vi "channelcontrolsub.vi"(0 "TorqueSample":dbl, 1 "dt":dbl, 3 "Limit Number":dbl, 4 "Torque":bool, 5 "ControlPara":dbl[](array[numeric]), 7 "AngleSample":dbl, 8 "Angel":bool, 9 "syn-Error":dbl, 12 "Command":dbl, 15 "TempAngle":dbl, 16 "output range":cluster{"output high":dbl, "output low":dbl}, 17 "ChannelStatus":T1 items=["通道关", "位置通道", "加载通道"]) -> (19 "syn out":dbl, 20 "output":dbl, 22 "forward":dbl, 23 "TempAngleOut":dbl, 24 "diff syn out 2":dbl, 25 "control out":dbl, 27 "Commandout":dbl)   [LabVIEW 2014]
uses:
  Control 1.ctl
  <vilib>/Analysis/3filter.llb/Filter Passband Type.ctl
  <vilib>/addons/control/pid/pid.llb/PID (DBL).vi
  <vilib>/addons/control/pid/NI_PID_pid.lvlib
  <vilib>/ptbypt/NI_PtbyPt.lvlib
  <vilib>/Analysis/NI_AALBase.lvlib
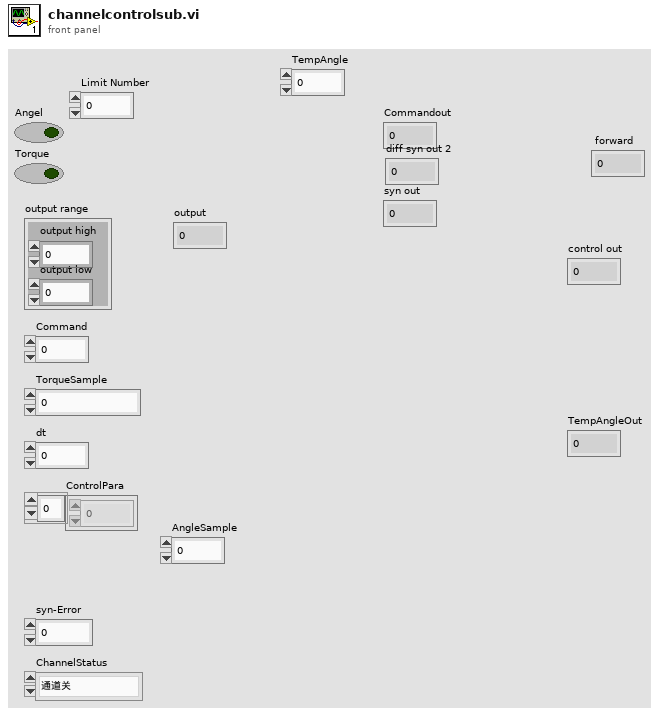
[diagram p1: front panel]
types:
  T1 = typedef "Control 1.ctl" = i32
  T2 = typedef "NI_AALBase.lvlib/Filter Passband Type.ctl" = enum32{"Lowpass", "Highpass", "Bandpass", "Bandstop"}
  T3 = cluster{"Numeric":dbl, "Numeric":dbl, "Numeric":dbl}
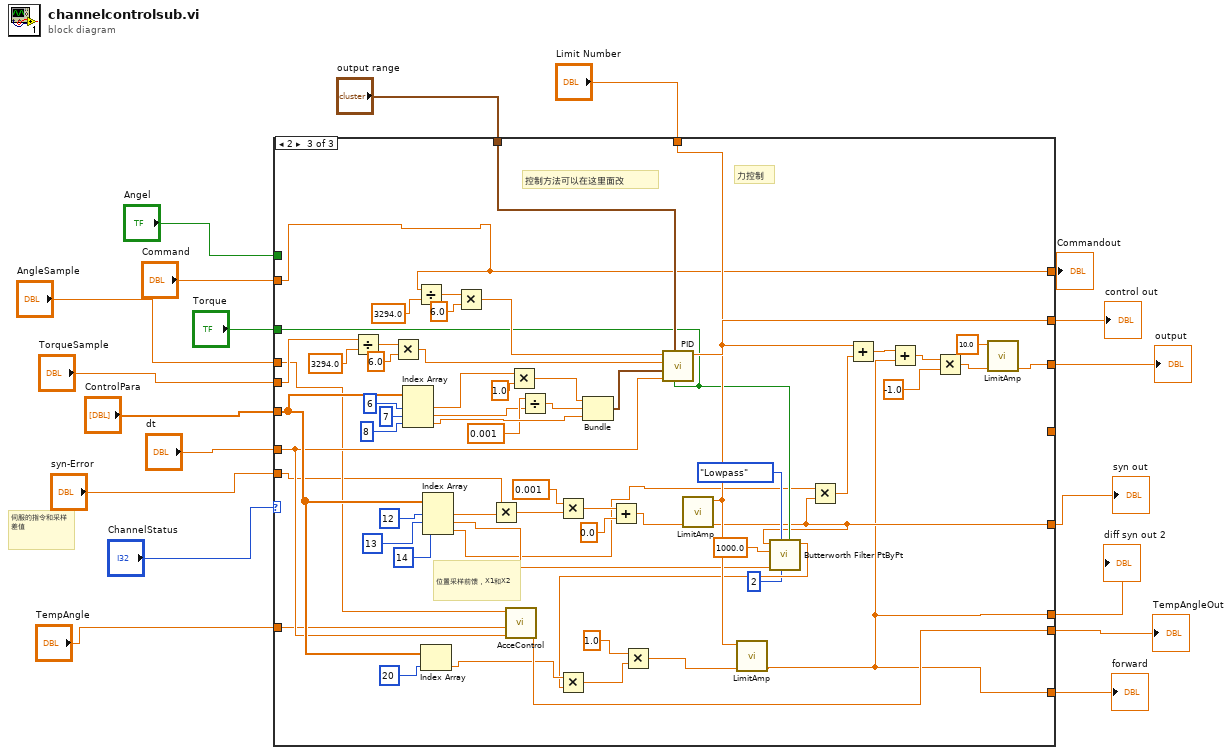
[diagram p0: block diagram]
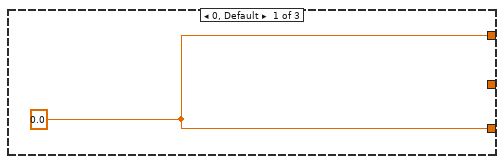
[diagram p2: hidden frame]
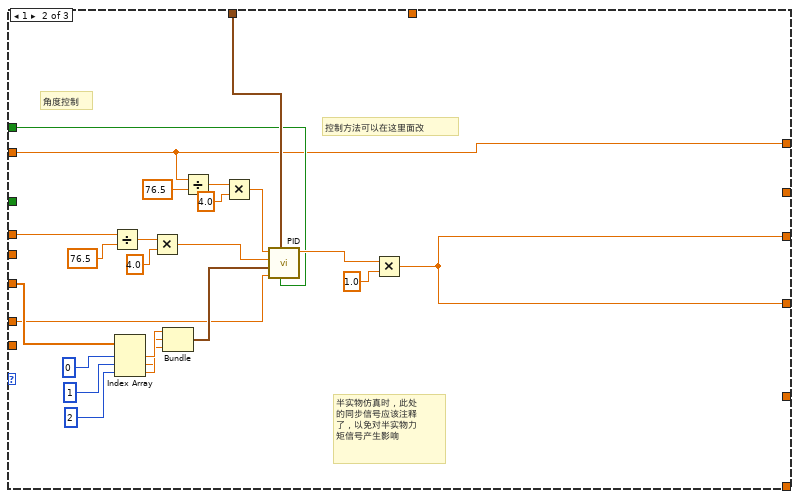
[diagram p3: hidden frame]
diagram:
  # "伺服的指令和采样差值"
  n1 = case shown="2" "ChannelStatus" {
    tunnel: "dt" -> [_ w29 w71]
    tunnel: "output range" -> [_ w26 w104]
    tunnel: "Command" -> [_ w21 w68]
    tunnel: "ControlPara" -> [_ w41 w80]
    tunnel: [w20 w24 w48] -> w18
    tunnel: "TorqueSample" -> [_ _ w89]
    tunnel: "syn-Error" -> [_ _ w67]
    tunnel: [_ w24 _] -> _
    tunnel: "AngleSample" -> [_ w23 w70]
    tunnel: "Angel" -> [_ w22 _]
    tunnel: "Torque" -> [_ _ w60]
    tunnel: [w20 w21 w68] -> w9
    tunnel: "TempAngle" -> [_ _ w69]
    tunnel: [_ _ w85] -> w8
    tunnel: [_ _ w82] -> w7
    tunnel: "Limit Number" -> [_ _ w78]
    tunnel: [_ _ w52] -> w2
    tunnel: [_ _ w46] -> w1
    tunnel: [_ _ w46] -> w5
    frame 0, Default {
      w20 = 0.0 ("output")
    }
    frame 1 {
      # "半实物仿真时，此处\n的同步信号应该注释\n了，以免对半实物力\n矩信号产生影响"
      # "控制方法可以在这里面改"
      # "角度控制"
      n2 = Divide(x=w23, y=76.5) -> (x/y=w35:dbl)
      n3 = Index Array(array=w41, index #1=0 ("index"), index #2=1 ("index"), index #3=2 ("index")) -> (element #1=w33:dbl, element #2=w25:dbl, element #3=w32:dbl)
      n4 = Multiply(x=w35, y=4.0) -> (x*y=w28:dbl)
      n5 = Bundle("Numeric"=w33, "Numeric"=w25, "Numeric"=w32) -> (w30:T3)  [unwired: 1 in]
      n6 = Divide(x=w21, y=76.5) -> (x/y=w38:dbl)
      n7 = Multiply(x=w38, y=4.0) -> (x*y=w27:dbl)
      n8 = call-poly <vilib>:"PID.vi"("reinitialize? (F)"=w22, "output range"=w26, "dt (s)"=w29, "PID gains"=w30, "process variable"=w28, "setpoint"=w27) -> ("output"=w31:dbl)  [unwired: 4 in, 1 out]
      n9 = Multiply(x=w31, y=1.0) -> (x*y=w24:dbl)
    }
    frame 2 {
      # "位置采样前馈，X1和X2"
      # "力控制"
      # "控制方法可以在这里面改"
      n10 = Divide(x=w89, y=3294.0) -> (x/y=w93:dbl)
      n11 = Multiply(x=w93, y=6.0) -> (x*y=w92:dbl)
      n12 = Index Array(array=w80, index #1=6 ("index"), index #2=7 ("index"), index #3=8 ("index")) -> (element #1=w74:dbl, element #2=w72:dbl, element #3=w91:dbl)
      n13 = Divide(x=w68, y=3294.0) -> (x/y=w97:dbl)
      n14 = Index Array(array=w80, index=20) -> (element=w66:dbl)
      n15 = Index Array(array=w80, index #1=12 ("index"), index #2=13 ("index"), index #3=14 ("索引")) -> (element #1=w65:dbl, element #2=w58:dbl, element #3=w50:dbl)
      n16 = Multiply(x=w97, y=6.0) -> (x*y=w96:dbl)
      n17 = Multiply(x=w67, y=w65) -> (x*y=w79:dbl)
      n18 = call "AcceControl.vi"("dt"=w71, "TempAngle"=w69, "angle sample"=w70) -> ("temp angle out"=w85:dbl)  [unwired: 7 in, 1 out]
      n19 = Multiply(x=w74, y=1.0) -> (x*y=w87:dbl)
      n20 = Divide(x=0.001 ("y"), y=w72) -> (x/y=w86:dbl)
      n21 = Multiply(x=0.001 ("y"), y=w79) -> (x*y=w63:dbl)
      n22 = Bundle(w87, w86, "Numeric"=w91) -> (w100:cluster{dbl, dbl, "Numeric":dbl})  [unwired: 1 in]
      n23 = Add(x=w63, y=0.0 ("x")) -> (x+y=w53:dbl)
      n24 = call-poly <vilib>:"PID.vi"("reinitialize? (F)"=w60, "output range"=w104, "dt (s)"=w71, "PID gains"=w100, "process variable"=w92, "setpoint"=w96) -> ("output"=w82:dbl)  [unwired: 4 in, 1 out]
      n25 = call "LimitAmp.vi"("data in"=w53, "limit"=w78) -> ("data out"=w52:dbl)  [unwired: 9 in]
      n26 = call <vilib>:"Butterworth Filter PtByPt.vi"("initialize"=w60, "order"=2, "filter type"=Filter_Passband_Type."Lowpass", "low cutoff freq: fl"=w58, "sampling freq: fs"=1000.0, "x"=w52) -> ("Filtered x"=w54:dbl)  [unwired: 3 in, 1 out]
      n27 = Multiply(x=w66, y=w54) -> (x*y=w55:dbl)
      n28 = Multiply(x=1.0 ("y"), y=w55) -> (x*y=w56:dbl)
      n29 = call "LimitAmp.vi"("data in"=w56, "limit"=w78) -> ("data out"=w46:dbl)  [unwired: 9 in]
      n30 = Multiply(x=w50, y=w52) -> (x*y=w51:dbl)
      n31 = Add(x=w82, y=w51) -> (x+y=w77:dbl)
      n32 = Add(x=w77, y=w46) -> (x+y=w76:dbl)
      n33 = Multiply(x=w76, y=-1.0) -> (x*y=w49:dbl)
      n34 = call "LimitAmp.vi"("data in"=w49, "limit"=10.0) -> ("data out"=w48:dbl)  [unwired: 9 in]
    }
  }
  "output" <- w18
  "Commandout" <- w9
  "syn out" <- w2
  "TempAngleOut" <- w8
  "control out" <- w7
  "forward" <- w1
  "diff syn out 2" <- w5
